vi "Joint Reference Follower.vi"(6 "Accurus Ctrl Cluster":T2={"Stop Accurus"=TRUE, "Vacuum Force"=0, "Max Limit [mmHg]"=600.0, "Slide in"=0} {"Slide in" scale=0.0..78.0; "Vacuum Force" min=0 max=78}, 7 "Offset Home2RCM [deg/mm]":dbl[](array[numeric])=[0.0, 0.0, 0.0, 0.0], 8 "PID Ctrl Cluster":T3={"L1 PID Gains"={"Kp"=0.005, "Kd"=0.5, "Ki"=0.0005}, "L2 PID Gains"={"Kp"=0.01, "Kd"=1.0, "Ki"=0.005}, "L3 PID Gains"={"Kp"=0.05, "Kd"=1.0, "Ki"=0.0005}, "L4 PID Gains"={"Kp"=0.1, "Kd"=0.1, "Ki"=0.0005}}, 9 "Ref Array [deg/mm]":dbl[](array[numeric])=[0.0, 0.0, 0.0, 0.0], 10 "error in":errorcluster, 11 "FPGA VI Reference In":refnum<k20>) -> (0 "Accurus Output Cluster":T1={"Vacuum Engaged?"=FALSE, "Voltage Ouptut Ch. A"=600.0, "Voltage Ouptut Ch. B"=600.0, "Vacuum Force [mmHg]"=600, "Foot Paddle 3"=600.0}, 1 "Output Posit Array [deg/mm]":dbl[](array[numeric]), 2 "error out":errorcluster, 3 "FPGA VI Reference Out":refnum<k20>)   [LabVIEW 2016]
uses:
  Subsystems/Global Variables v1.vi
  <vilib>/Utility/error.llb/Error Cluster From Error Code.vi
  <vilib>/rvi/errors/niLvFpgaAdjustHostInterfaceError.vi
  <vilib>/rvi/interface/nirviReadWriteControl/nirviReadWriteControl.xnode
  FPGA Bitfiles/PhantomControlPI_FPGATarget_QuadCtr2_E2412E44.lvbitx
  IRISS_FPGA_IO.vi
  Library/KevinLibraryAll/labview/KevLib01.lvlib
  NiFpgaLv.dll
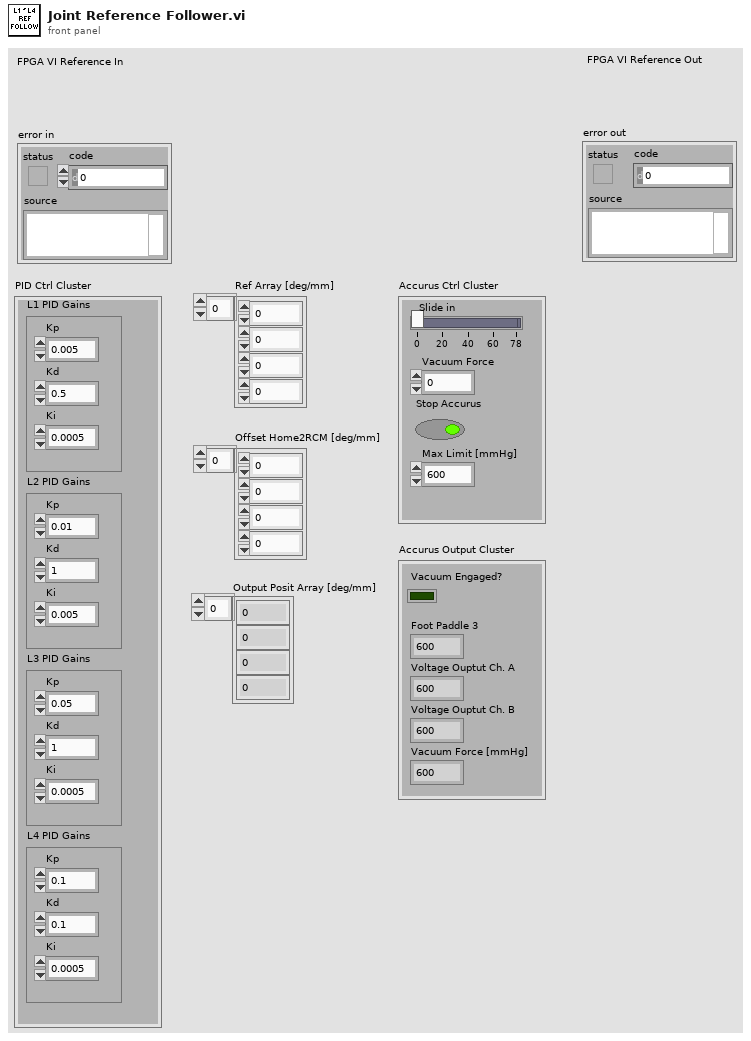
[diagram p1: front panel]
types:
  T1 = cluster{"Vacuum Engaged?":bool, "Voltage Ouptut Ch. A":dbl, "Voltage Ouptut Ch. B":dbl, "Vacuum Force [mmHg]":i32, "Foot Paddle 3":dbl}
  T2 = cluster{"Stop Accurus":bool, "Vacuum Force":i8, "Max Limit [mmHg]":dbl, "Slide in":i8}
  T3 = cluster{"L1 PID Gains":cluster{"Kp":dbl, "Kd":dbl, "Ki":dbl}, "L2 PID Gains":cluster{"Kp":dbl, "Kd":dbl, "Ki":dbl}, "L3 PID Gains":cluster{"Kp":dbl, "Kd":dbl, "Ki":dbl}, "L4 PID Gains":cluster{"Kp":dbl, "Kd":dbl, "Ki":dbl}}
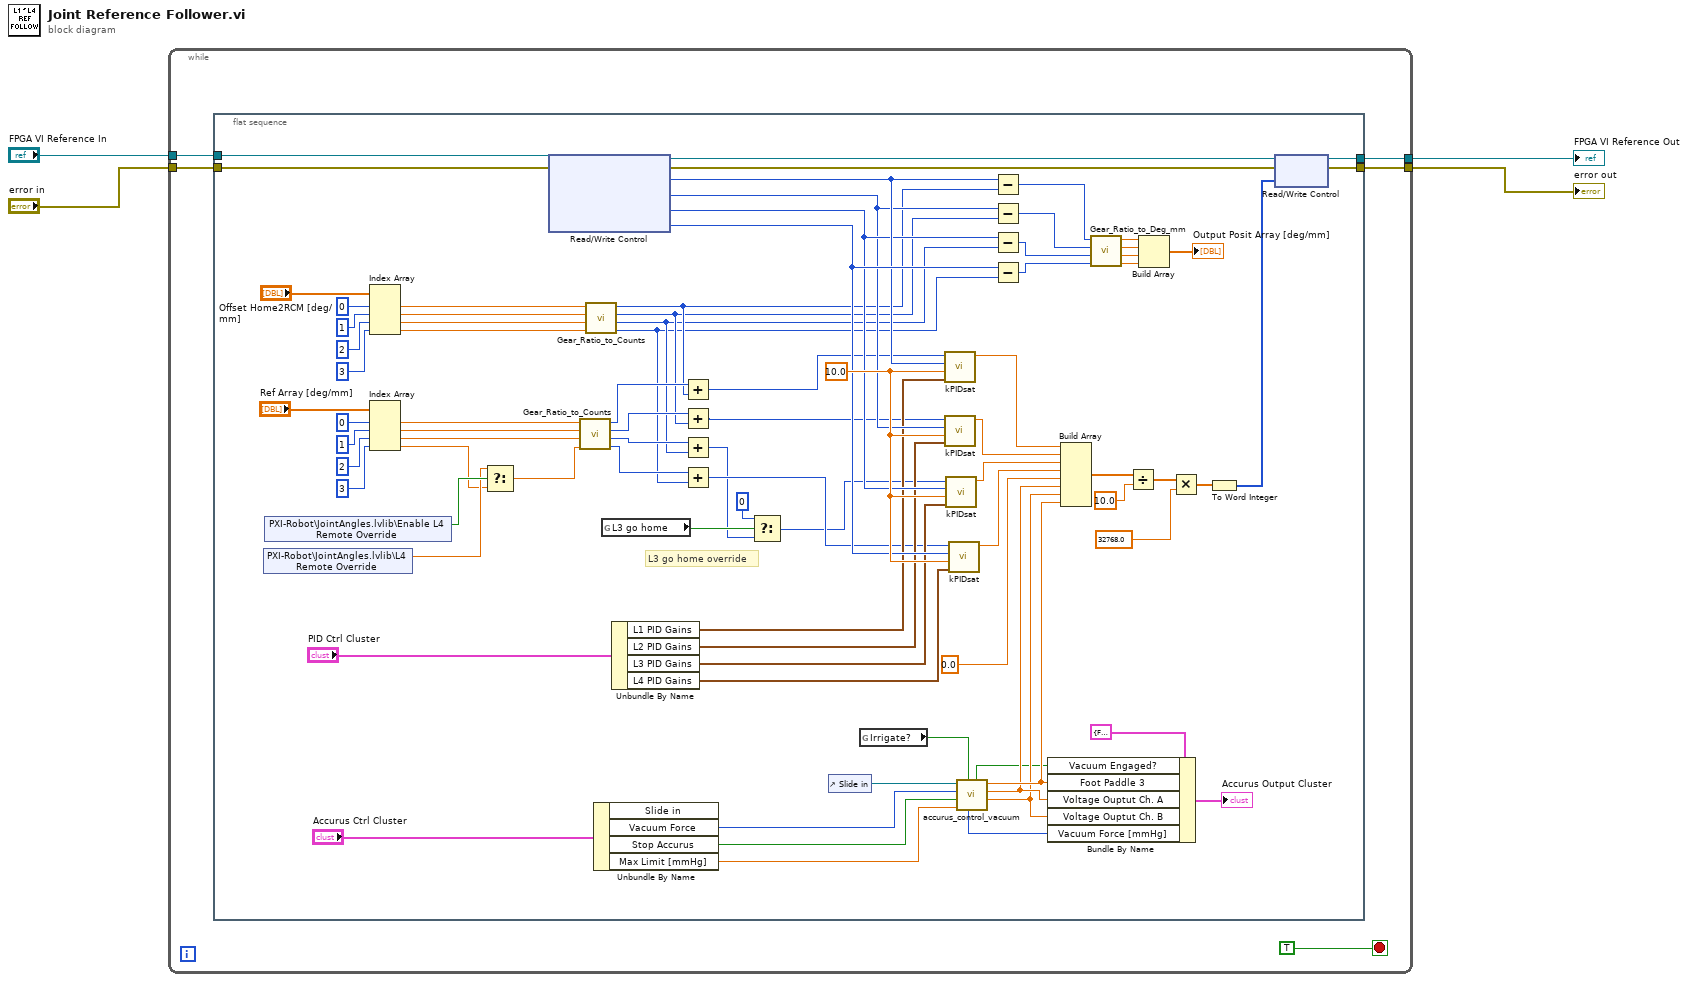
[diagram p0: block diagram]
diagram:
  n1 = while {
    tunnel: [w9] -> w4
    tunnel: [w8] -> w3
    tunnel: "FPGA VI Reference In" -> [w7]
    tunnel: "error in" -> [w6]
    stop <- TRUE ("Boolean") stop-if-true
    n2 = flat-sequence {
      tunnel: [w70] -> w9
      tunnel: [w69] -> w8
      tunnel: w7 -> [w44]
      tunnel: w6 -> [w43]
      frame #0 {
        w80 = 10.0 ("Sat Limit")
        # "L3 go home override"
        n3 = shared-variable "PXI-Robot\\JointAngles.lvlib\\L4 Remote Override"() -> (w13:dbl)  [unwired: 1 in, 1 out]
        n4 = shared-variable "PXI-Robot\\JointAngles.lvlib\\Enable L4 Remote Override"() -> (w15:bool)  [unwired: 1 in, 1 out]
        n5 = Index Array(array="Offset Home2RCM [deg/mm]", index #1=0 ("index"), index #2=1 ("index"), index #3=2 ("index"), index #4=3 ("index")) -> (element #1=w42:dbl, element #2=w41:dbl, element #3=w40:dbl, element #4=w39:dbl)
        n6 = Index Array(array="Ref Array [deg/mm]", index #1=0 ("index"), index #2=1 ("index"), index #3=2 ("index"), index #4=3 ("index")) -> (element #1=w88:dbl, element #2=w87:dbl, element #3=w86:dbl, element #4=w12:dbl)
        n7 = Select(t=w13, s=w15, f=w12) -> (s? t:f=w14:dbl)
        n8 = xnode "Read/Write Control"("FPGA VI Reference In"=w44, "error in"=w43) -> ("FPGA VI Reference Out"=w72:refnum<k20>, "error out"=w71:errorcluster, "32 bit Position 1"=w51:i32, "32 bit Position 3"=w49:i32, "32 bit Position C1-1"=w50:i32, "32 bit Position C1-4"=w61:i32)
        n9 = call "Gear_Ratio_to_Counts.vi"("theta 4"=w14, "theta 3"=w86, "theta 2"=w87, "theta 1"=w88) -> ("j4"=w32:i32, "j3"=w33:i32, "j2"=w34:i32, "j1"=w35:i32)
        n10 = call "Gear_Ratio_to_Counts.vi"("theta 4"=w39, "theta 3"=w40, "theta 2"=w41, "theta 1"=w42) -> ("j4"=w28:i32, "j3"=w29:i32, "j2"=w30:i32, "j1"=w31:i32)
        n11 = Unbundle By Name("Accurus Ctrl Cluster") -> ("Vacuum Force"=w26:i8, "Stop Accurus"=w25:bool, "Max Limit [mmHg]"=w24:dbl)  [unwired: 1 out]
        n12 = global read "Global Variables v1.vi" "L3 go home"() -> (w19:bool)
        n13 = Unbundle By Name("PID Ctrl Cluster") -> ("L1 PID Gains"=w48:cluster{"Kp":dbl, "Kd":dbl, "Ki":dbl}, "L2 PID Gains"=w47:cluster{"Kp":dbl, "Kd":dbl, "Ki":dbl}, "L3 PID Gains"=w46:cluster{"Kp":dbl, "Kd":dbl, "Ki":dbl}, "L4 PID Gains"=w45:cluster{"Kp":dbl, "Kd":dbl, "Ki":dbl})
        n14 = Add(x=w35, y=w31) -> (x+y=w38:i32)
        n15 = Add(x=w34, y=w30) -> (x+y=w37:i32)
        n16 = Add(x=w33, y=w29) -> (x+y=w18:i32)
        n17 = Add(x=w32, y=w28) -> (x+y=w36:i32)
        n18 = Select(t=0 ("index"), s=w19, f=w18) -> (s? t:f=w16:i32)
        n19 = control-ref of="Slide in"() -> (w23:refnum<vi>)
        n20 = global read "Global Variables v1.vi" "Irrigate?"() -> (w10:bool)
        n21 = call "kPIDsat.vi"("PID Gains"=w48, "Sat Limit"=w80, "Position"=w51, "Reference"=w38) -> ("Control"=w60:dbl)  [unwired: 7 in]
        n22 = call "kPIDsat.vi"("PID Gains"=w47, "Sat Limit"=w80, "Position"=w49, "Reference"=w37) -> ("Control"=w62:dbl)  [unwired: 7 in]
        n23 = call "kPIDsat.vi"("PID Gains"=w46, "Sat Limit"=w80, "Position"=w50, "Reference"=w16) -> ("Control"=w63:dbl)  [unwired: 7 in]
        n24 = call "kPIDsat.vi"("PID Gains"=w45, "Sat Limit"=w80, "Position"=w61, "Reference"=w36) -> ("Control"=w79:dbl)  [unwired: 7 in]
        n25 = call "accurus_control_vacuum.vi"("Irrigate?"=w10, "Max Limit [mmHg]"=w24, "stop"=w25, "vacuum force"=w26, "Slide in"=w23) -> ("f"=w65:dbl, "f 2"=w66:dbl, "f 3"=w67:dbl, "Boolean 2"=w22:bool, "Vacuum Force\n[mmHg]"=w20:i32)  [unwired: 1 in, 1 out]
        n26 = Subtract(x=w51, y=w31) -> (x-y=w55:i32)
        n27 = Subtract(x=w49, y=w30) -> (x-y=w54:i32)
        n28 = Subtract(x=w50, y=w29) -> (x-y=w53:i32)
        n29 = Subtract(x=w61, y=w28) -> (x-y=w52:i32)
        n30 = Bundle By Name(cluster=T1 {"Vacuum Engaged?"=FALSE, "Voltage Ouptut Ch. A"=0.0, "Voltage Ouptut Ch. B"=0.0, "Vacuum Force [mmHg]"=0, "Foot Paddle 3"=0.0} ("Accurus Output Cluster 2"), "Vacuum Engaged?"=w22, "Foot Paddle 3"=w67, "Voltage Ouptut Ch. A"=w66, "Voltage Ouptut Ch. B"=w65, "Vacuum Force [mmHg]"=w20) -> (→"Accurus Output Cluster":T1)
        n31 = Build Array(w60, w62, w63, w79, 0.0 ("element"), w66, w65, w67) -> (w78:dbl[])
        n32 = call "Gear_Ratio_to_Deg_mm.vi"("j4"=w52, "j3"=w53, "j2"=w54, "j1"=w55) -> ("theta 4"=w56:dbl, "theta 3"=w57:dbl, "theta 2"=w58:dbl, "theta 1"=w59:dbl)
        n33 = Divide(x=w78, y=10.0) -> (x/y=w76:dbl[])
        n34 = Build Array(w59, w58, w57, w56) -> (→"Output Posit Array [deg/mm]":dbl[])
        n35 = Multiply(x=w76, y=32768.0) -> (x*y=w74:dbl[])
        n36 = To Word Integer(number=w74) -> (16bit integer=w73:i16[])
        n37 = xnode "Read/Write Control"("FPGA VI Reference In"=w72, "error in"=w71, "AO"=w73) -> ("FPGA VI Reference Out"=w70:refnum<k20>, "error out"=w69:errorcluster)
      }
    }
  }
  "FPGA VI Reference Out" <- w4
  "error out" <- w3
